vi "KH7008 COM.vi"(8 "error in (no error)":errorcluster, 10 "Command":string, 11 "VISA Refnum in":refnum<visa-resource-name>="COM3") -> (0 "error out":errorcluster, 2 "Response":string="\r\n", 3 "VISA Refnum out":refnum<visa-resource-name>)   [LabVIEW 2019, in "Instrument.KH7008.lvclass"]
uses:
  Instrument.KH7008.lvclass
  <vilib>/Instr/_visa.llb/VISA Configure Serial Port (Instr).vi
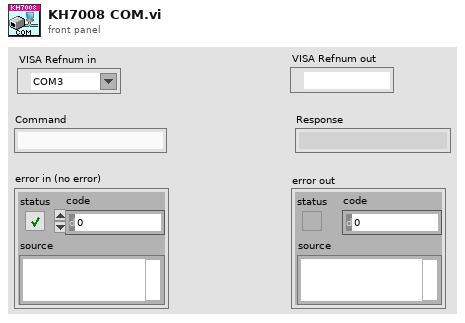
[diagram p1: front panel]
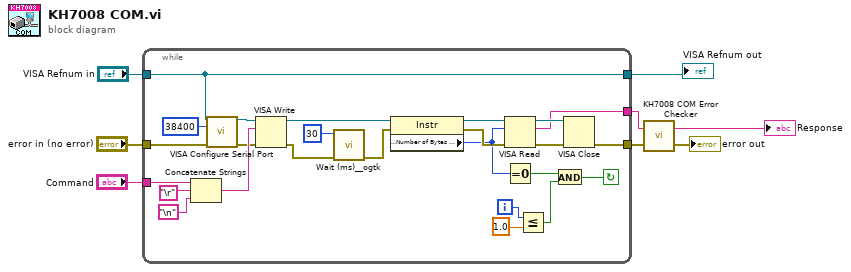
[diagram p0: block diagram]
diagram:
  n1 = while {
    tunnel: "VISA Refnum in" -> [w12]
    tunnel: "Command" -> [w23]
    tunnel: "error in (no error)" -> [w17]
    tunnel: [w16] -> w5
    tunnel: [w15] -> w2
    tunnel: [w12] -> w1
    i -> [w21]
    stop <- w18 continue-if-true
    n2 = Concatenate Strings(w23, "\r", "\n") -> (w33:string)
    n3 = call-poly "VISA Configure Serial Port"("VISA resource name"=w12, "baud rate (9600)"=u32 38400 ("baud rate"), "error in (no error)"=w17) -> ("VISA resource name out"=w30:refnum<visa-resource-name>, "error out"=w31:errorcluster)  [unwired: 6 in, 5 out]
    n4 = VISA Write(VISA resource name=w30, write buffer=w33, error in (no error)=w31) -> (VISA resource name out=w28:refnum<visa-resource-name>, error out=w27:errorcluster)  [unwired: 1 out]
    n5 = call <userlib>:"Wait (ms)__ogtk.vi"("error in (no error)"=w27, "milliseconds to wait"=u32 30) -> ("error out"=w13:errorcluster)  [unwired: 8 in, 1 out]
    n6 = property class="Instr"(reference=w28, error in=w13) -> (reference out=w29:refnum<visa-resource-name>, error out=w10:errorcluster, "Serial Settings:Number of Bytes at Serial Port"=w9:u32)
    n7 = VISA Read(VISA resource name=w29, byte count=w9, error in (no error)=w10) -> (VISA resource name out=w26:refnum<visa-resource-name>, read buffer=w15:string, error out=w25:errorcluster)  [unwired: 1 out]
    n8 = Equal To 0?(x=w9) -> (x = 0?=w20:bool)
    n9 = Less Or Equal?(x=w21, y=1.0) -> (x <= y?=w19:bool)
    n10 = And(x=w20, y=w19) -> (x .and. y?=w18:bool)
    n11 = VISA Close(VISA resource name=w26, error in (no error)=w25) -> (error out=w16:errorcluster)
  }
  "VISA Refnum out" <- w1
  n12 = call "KH7008 COM Error Checker.vi"("error in (no error)"=w5, "String In"=w2) -> ("error out"=→"error out":errorcluster, "String"=→"Response":string)
